vi "TransferData.vi"(0 "Fehler (Eingang, kein Fehler)":errorcluster, 5 "instanceHandle":u32, 7 "DLL-Path":path, 9 "maxValues":i32) -> (3 "read":i32, 4 "Fehler (Ausgang)":errorcluster, 6 "instanceHandle":u32, 8 "DLL-Path":path, 10 "ERR_CODE":i32, 14 "scaledData":dbl[](array[numeric]), 15 "rawData":i32[](array[numeric]))   [LabVIEW 2015, in "MEDAQLib.lvlib"]
doc: "ERR_CODE TransferData (DWORD instanceHandle, int *rawData, double *scaledData, int maxValues, int *read);\n\nTransfer the data from driver to application."
uses:
  MEDAQLib.lvlib
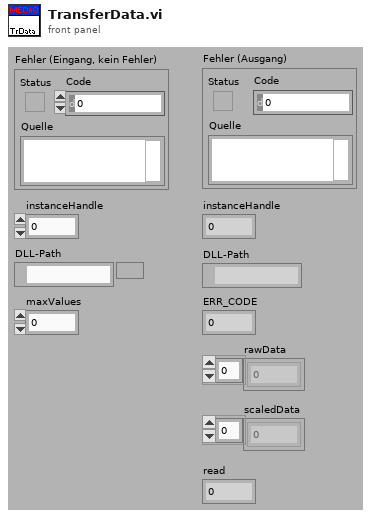
[diagram p1: front panel]
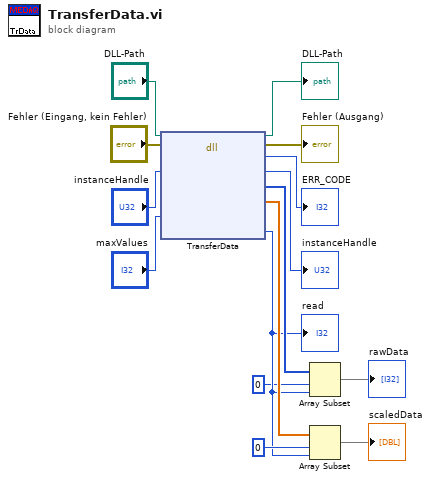
[diagram p0: block diagram]
diagram:
  n1 = dll-call lib="C:/Programme/National Instruments 8.6/LabVIEW 8.6/instr.lib/MEDAQLib/Release/MEDAQLib.dll" fn="TransferData"(path in="DLL-Path", error in="Fehler (Eingang, kein Fehler)", "instanceHandle"="instanceHandle", "maxValues"="maxValues") -> (path out=→"DLL-Path":path, error out=→"Fehler (Ausgang)":errorcluster, "Rückgabetyp"=→"ERR_CODE":i32, "instanceHandle"=→"instanceHandle":u32, "rawData"=w6:i32[], "scaledData"=w9:dbl[], "read"=w4:i32)  [unwired: 2 in, 3 out]
  "read" <- w4
  n2 = Array Subset(array=w6, index=0 ("Index"), length=w4) -> (→"rawData":i32[])
  n3 = Array Subset(array=w9, index=0 ("Index"), length=w4) -> (→"scaledData":dbl[])
